vi "create SimpleChecking.vi"(6 "Inital Amount (0)":dbl, 8 "error in (no error)":errorcluster, 9 "Routing Number":string, 10 "Account Number":string, 11 "SimpleChecking in":refnum<class "SimpleChecking.lvclass">) -> (0 "error out":errorcluster, 3 "SimpleChecking out":refnum<class "SimpleChecking.lvclass">)   [LabVIEW 2020, in "SimpleChecking.lvclass"]
uses:
  SimpleChecking.lvclass
  SimpleChecking.lvclass/SimpleChecking.ctl
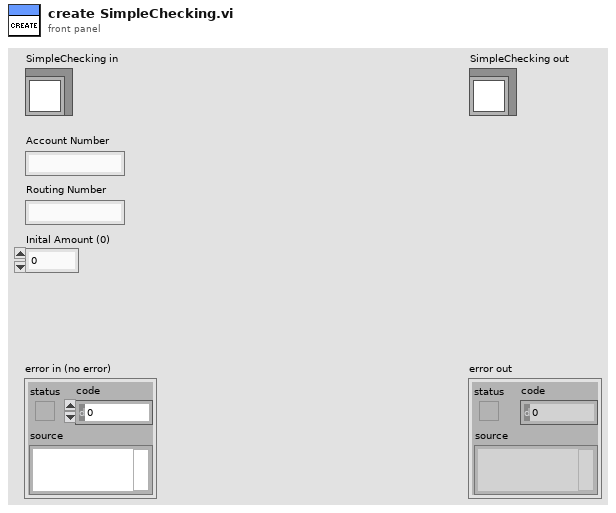
[diagram p1: front panel]
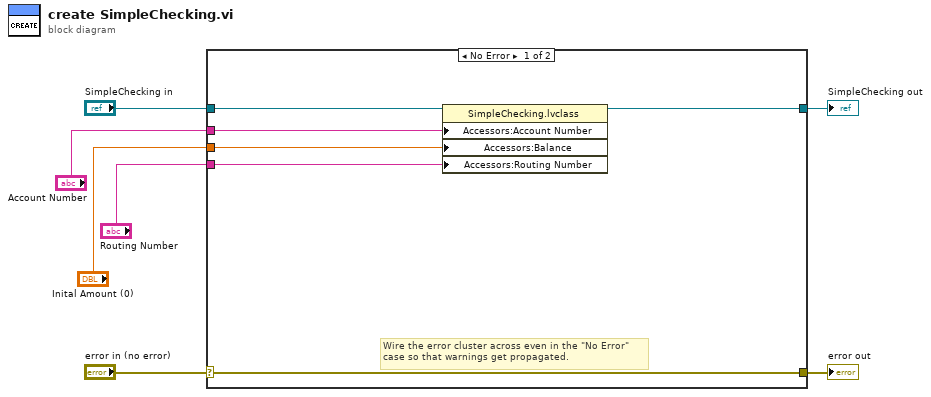
[diagram p0: block diagram]
diagram:
  n1 = case shown="No Error" "error in (no error)" {
    selector: "error in (no error)" -> [w12 w15]
    tunnel: [w12 w15] -> w6
    tunnel: [w11 w14] -> w4
    tunnel: "SimpleChecking in" -> [w13 w14]
    tunnel: "Account Number" -> [w10 _]
    tunnel: "Inital Amount (0)" -> [w9 _]
    tunnel: "Routing Number" -> [w8 _]
    frame No Error {
      # "Wire the error cluster across even in the \"No Error\"\ncase so that warnings get propagated."
      n2 = property class="SimpleChecking.lvclass"(reference=w13, "Accessors:Account Number"=w10, "Accessors:Balance"=w9, "Accessors:Routing Number"=w8) -> (reference out=w11:refnum<class "SimpleChecking.lvclass">)  [unwired: 1 in, 1 out]
    }
    frame Error {
    }
  }
  "error out" <- w6
  "SimpleChecking out" <- w4
